vi "kolejkaFIFO.vi"() -> ()   [LabVIEW 2018]
uses:
  <vilib>/sound2/lvsound2.llb/Sound Data Format.ctl
  lab6/stany.ctl
  <vilib>/sound2/lvsound2.llb/Sampling Mode.ctl
  <vilib>/sound2/lvsound2.llb/Sound Input Read (DBL).vi
panel:
  out "Waveform Graph":waveform(dbl)[](graph)
  in  "sound format":T1={"sample rate (S/s)"=22050.0, "number of channels"=2, "bits per sample"=16}
  in  "PLAY":bool
  out "Numeric":i32
  in  "number of samples/ch":i32=100000
  in  "?":bool
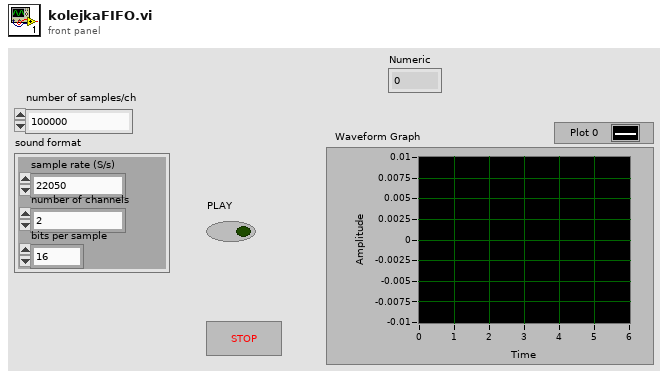
[diagram p1: front panel]
types:
  T1 = typedef "Sound Data Format.ctl" = cluster{"sample rate (S/s)":dbl, "number of channels":i32, "bits per sample":i32}
  T2 = typedef "stany.ctl" = enum16{"Indle", "Initialization", "Acquisition", "End"}
  T3 = typedef "Sampling Mode.ctl" = i32
  T4 = typedef "Sound Input Task ID.ctl" = u32
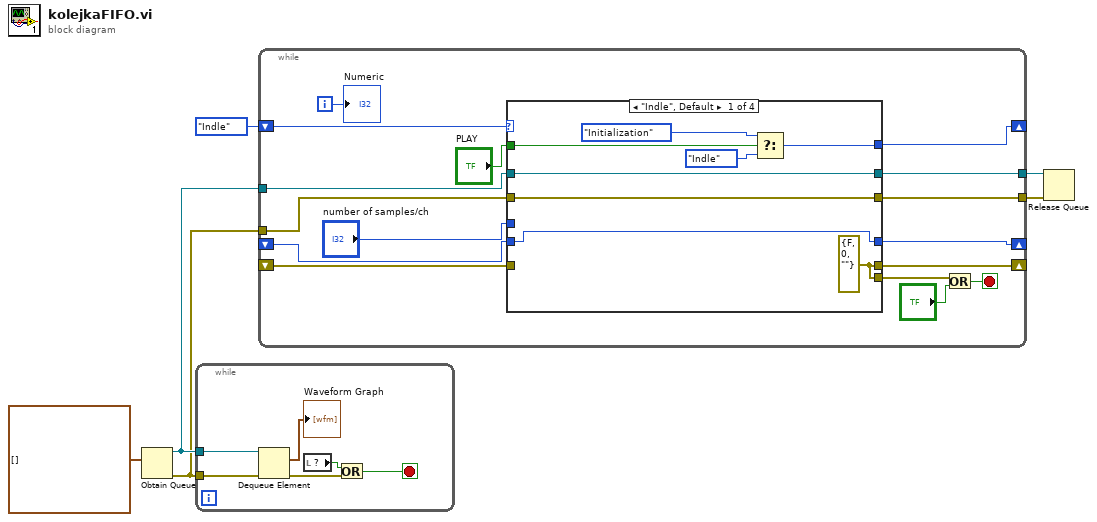
[diagram p0: block diagram]
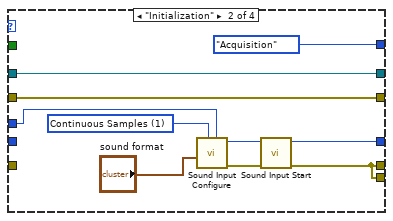
[diagram p2: hidden frame]
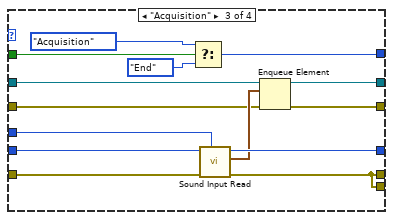
[diagram p3: hidden frame]
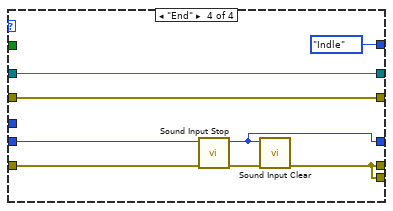
[diagram p4: hidden frame]
diagram:
  n1 = Obtain Queue(element data type=waveform(dbl)[] [] ("data")) -> (queue out=w3:refnum<queue>, error out=w2:errorcluster)  [unwired: 4 in, 1 out]
  n2 = while {
    tunnel: w3 -> [w12]
    tunnel: w2 -> [w11]
    stop <- w9 stop-if-true
    n3 = Dequeue Element(queue=w12, error in (no error)=w11) -> (element=→"Waveform Graph":waveform(dbl)[], error out=w7:errorcluster)  [unwired: 1 in, 2 out]
    n4 = local read item#?() -> (w8:bool)
    n5 = Or(x=w8, y=w7) -> (x .or. y?=w9:bool)
  }
  n6 = while {
    shift-right: [w27] -> _
    shift-left: stany."Indle" -> [w28]
    shift-right: [w24] -> _
    shift-left: _ -> [w23]
    shift-right: [w25] -> _
    shift-left: _ -> [w22]
    tunnel: w2 -> [w17]
    tunnel: [w16] -> w5
    tunnel: [w15] -> w4
    tunnel: w3 -> [w14]
    i -> [w21]
    stop <- w18 stop-if-true
    n7 = case shown="\"Indle\", Default" w28 {
      tunnel: [w34 stany."Acquisition" w57 stany."Indle"] -> w27
      tunnel: "PLAY" -> [w33 _ w60 _]
      tunnel: [w32 w43 w54 w64] -> w25
      tunnel: [w31 w39 w52 w63] -> w24
      tunnel: w23 -> [_ _ w55 w66]
      tunnel: w22 -> [w32 _ w56 w65]
      tunnel: "number of samples/ch" -> [_ w40 w53 _]
      tunnel: [w31 w39 w52 w63] -> w19
      tunnel: w17 -> [w29 w37 w50 w61]
      tunnel: [w29 w37 w49 w61] -> w16
      tunnel: [w30 w38 w48 w62] -> w15
      tunnel: w14 -> [w30 w38 w47 w62]
      frame "Indle", Default {
        w31 = errorcluster {"status"=FALSE, "code"=0, "source"=""} ("error out")
        n8 = Select(t=stany."Initialization", s=w33, f=stany."Indle") -> (s? t:f=w34:T2)
      }
      frame "Initialization" {
        w41 = T3 1 items=["Finite Samples", "Continuous Samples"] ("sample mode")
        n9 = call <vilib>:"Sound Input Configure.vi"("number of samples/ch"=w40, "sample mode"=w41, "sound format"="sound format") -> ("error out"=w45:errorcluster, "task ID"=w46:T4)  [unwired: 7 in]
        n10 = call <vilib>:"Sound Input Start.vi"("error in (no error)"=w45, "task ID"=w46) -> ("error out"=w39:errorcluster, "task ID out"=w43:T4)  [unwired: 8 in]
      }
      frame "Acquisition" {
        n11 = Select(t=stany."Acquisition", s=w60, f=stany."End") -> (s? t:f=w57:T2)
        n12 = call-poly <vilib>:"Sound Input Read.vi"("number of samples/ch"=w53, "error in (no error)"=w55, "task ID"=w56) -> ("error out"=w52:errorcluster, "data"=w51:waveform(dbl)[], "task ID out"=w54:T4)  [unwired: 6 in]
        n13 = Enqueue Element(queue=w47, element=w51, error in (no error)=w50) -> (queue out=w48:refnum<queue>, error out=w49:errorcluster)  [unwired: 1 in, 1 out]
      }
      frame "End" {
        n14 = call <vilib>:"Sound Input Stop.vi"("error in (no error)"=w66, "task ID"=w65) -> ("error out"=w68:errorcluster, "task ID out"=w64:T4)  [unwired: 8 in]
        n15 = call <vilib>:"Sound Input Clear.vi"("error in (no error)"=w68, "task ID"=w64) -> ("error out"=w63:errorcluster)  [unwired: 9 in]
      }
    }
    n16 = Or(x=w19, y="?") -> (x .or. y?=w18:bool)
    "Numeric" <- w21
  }
  n17 = Release Queue(queue=w4, error in (no error)=w5) -> ()  [unwired: 1 in, 3 out]
